vi "Delete Notebook Backup on Quit.vi"(8 "Error In":errorcluster, 11 "Main VI Name":string) -> (0 "Error Out":errorcluster)   [LabVIEW 2019, in "Notebook.lvlib"]
uses:
  Notebook.lvlib
panel:
  # "Check if the Notebook window is open:\nif it is,  don'r do anything.\nif it isn't, delete the backup.\n\nCall this VI when quitting your application."
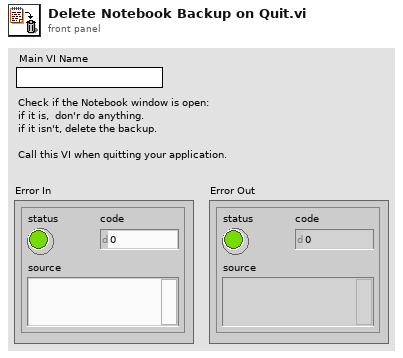
[diagram p1: front panel]
types:
  T1 = enum32{"Invalid", "Standard", "Closed", "Hidden", "Minimized", "Maximized"}
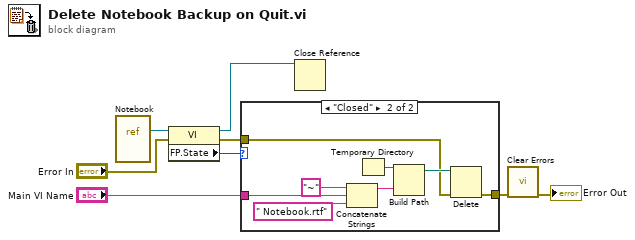
[diagram p0: block diagram]
diagram:
  n1 = vi-ref "Notebook.vi"() -> (w8:refnum<vi>)
  n2 = property class="VI"(reference=w8, error in="Error In") -> (reference out=w5:refnum<vi>, error out=w6:errorcluster, "FP.State"=w7:T1)
  n3 = case shown="\"Closed\"" w7 {
    tunnel: "Main VI Name" -> [_ w13]
    tunnel: w6 -> [w9 w11]
    tunnel: [w9 w10] -> w4
    frame "Invalid", Default {
    }
    frame "Closed" {
      n4 = Concatenate Strings("~" ("string"), w13, " Notebook.rtf" ("format string")) -> (w14:string)
      n5 = Temporary Directory() -> (w17:path)
      n6 = Build Path(base path=w17, name or relative path=w14) -> (appended path=w12:path)
      n7 = Delete(path (use dialog)=w12, error in=w11) -> (error out=w10:errorcluster)  [unwired: 3 in, 2 out]
    }
  }
  n8 = Close Reference(reference=w5) -> ()  [unwired: 1 in, 1 out]
  n9 = call <vilib>:"Clear Errors.vi"("error in (no error)"=w4) -> ("error out"=→"Error Out":errorcluster)  [unwired: 5 in, 1 out]
